vi "Begin.vi"(8 "error in":errorcluster) -> (0 "error out":errorcluster)   [LabVIEW 2017]
doc: "Called before other user functions, this VI is expected to open initial I/O refnums, load in file data, and do all program initialization. Notice that the <B>error out</B> terminal is simply used for data flow. Wiring it to other structures or subVIs ensures that this VI runs first."
uses:
  <vilib>/Rock Robotics/WPI/SafetyOutput/WPI_SafetyOutputConfigMenu.ctl
  <vilib>/Rock Robotics/WPI/Joystick/WPI_JoystickDeviceEnum.ctl
  <vilib>/Rock Robotics/WPI/DriverStation/WPI_DriverStationRobotMode2.ctl
  <vilib>/Rock Robotics/WPI/Solenoid/WPI_SolenoidChannel.ctl
  <vilib>/Rock Robotics/WPI/ThirdParty/Phoenix-LabVIEW/Motor Controller/Controls/CTRE_Phoenix_MotorControl_NeutralMode.ctl
  <vilib>/Rock Robotics/SystemInterfaces/DIO/FPGA_DIOChannel.ctl
  <vilib>/Rock Robotics/WPI/Solenoid/WPI_SolenoidValue.ctl
  <vilib>/Rock Robotics/Network Tables/NT Write String Array.vi
  <vilib>/Rock Robotics/WPI/Solenoid/WPI_SolenoidOpenDouble.vi
  Robot Global Data.vi
  <vilib>/Rock Robotics/WPI/Solenoid/WPI_SolenoidSetEnum.vi
  <vilib>/Rock Robotics/WPI/Counter/WPI_CounterDigitalInputToDigitalSource.vi
  <vilib>/Rock Robotics/WPI/ThirdParty/Phoenix-LabVIEW/Pigeon IMU/CTRE_PigeonIMU_Open_TalonSRX.vi
  <vilib>/Rock Robotics/WPI/RobotDrive/WPI_RobotDriveOpen2MotorWithExistingMotors.vi
  <vilib>/Rock Robotics/WPI/RobotDrive/WPI_RobotDriveOpen4MotorWithExistingMotors.vi
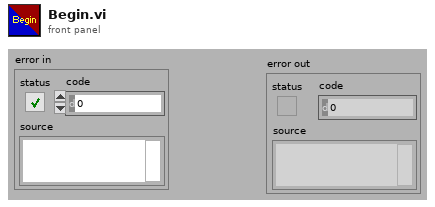
[diagram p1: front panel]
types:
  T1 = typedef "WPI_SolenoidValue.ctl" = enum16{"Off", "On", "Forward", "Reverse"}
  T2 = typedef "WPI_SolenoidChannel.ctl" = enum8{"Solenoid 0", "Solenoid 1", "Solenoid 2", "Solenoid 3", "Solenoid 4", "Solenoid 5", "Solenoid 6", "Solenoid 7", "Invalid"}
  T3 = typedef "FPGA_DIOChannel.ctl" = enum8{"DIO 0", "DIO 1", "DIO 2", "DIO 3", "DIO 4", "DIO 5", "DIO 6", "DIO 7", "DIO 8", "DIO 9", "DIO MXP 0", "DIO MXP 1", "DIO MXP 2", "DIO MXP 3", "DIO MXP 4", "DIO MXP 5", "DIO MXP 6", "DIO MXP 7", "DIO MXP 8", "DIO MXP 9", "DIO MXP 10", "DIO MXP 11", "DIO MXP 12", "DIO MXP 13", "DIO MXP 14", "DIO MXP 15", "SPI Port CS1", "SPI Port CS2", "SPI Port CS3", "SPI Port MISO", "SPI Port MOSI", "Invalid"}
  T4 = typedef "CTRE_Phoenix_MotorControl_NeutralMode.ctl" = enum8{"EEPROMSetting", "Override to Coast", "Override to Brake"}
  T5 = typedef "WPI_JoystickDeviceEnum.ctl" = enum16{"USB 0", "USB 1", "USB 2", "USB 3", "USB 4", "USB 5"}
  T6 = typedef "WPI_DriverStationRobotMode2.ctl" = enum16{"Autonomous Disabled", "Autonomous Enabled", "Teleop Disabled", "Teleop Enabled", "Disconnected", "Finish", "Test Disabled", "Test Enabled", "Emergency Stopped"}
  T7 = typedef "WPI_SafetyOutputConfigMenu.ctl" = enum16{"Enable", "Disable"}
  T8 = enum16{"FollowerType_PercentOutput", "FollowerType_AuxOutput1"}
  T9 = typedef "WPI_MotorControlDeviceRef.ctl" = cluster{"DeviceStatus":errorcluster, "Type":T10, "PWM":cluster{"PWM Channel":T11, "DeadBand":T12}, "CAN":cluster{"Device Number":u8, "SetOutput VI Ref":variant, "GetOutput VI Ref":variant, "Enable VI Ref":variant, "Disable VI Ref":variant, "Data":variant}, "Invert":bool, "DIO PWM":cluster{"PWM \"Enable\" Channel":T11, "DIOChannel":T3, "PWM Rate":dbl}}
  T10 = typedef "WPI_MotorControlType.ctl" = enum16{"PWM", "CAN", "DIO PWM"}
  T11 = typedef "FPGA_DIOPWMChannel.ctl" = enum8{"PWM 0", "PWM 1", "PWM 2", "PWM 3", "PWM 4", "PWM 5", "PWM 6", "PWM 7", "PWM 8", "PWM 9", "PWM MXP 0", "PWM MXP 1", "PWM MXP 2", "PWM MXP 3", "PWM MXP 4", "PWM MXP 5", "PWM MXP 6", "PWM MXP 7", "PWM MXP 8", "PWM MXP 9", "Invalid"}
  T12 = typedef "WPI_PWMDeadband.ctl" = cluster{"Name":string, "maxPositivePwm":i32, "minPositivePwm":i32, "centerPwm":i32, "maxNegativePwm":i32, "minNegativePwm":i32, "angularRange":u16}
  T13 = typedef "CTRE_PigeonIMU_DeviceRef.ctl" = cluster{"DeviceStatus":errorcluster, "Device Number":u8, "Type":T14, "Device ID":u32, "Handle":u64, "UsageFrame":u32, "Library Path":path}
  T14 = typedef "CTRE_PigeonIMU_ConnectionType.ctl" = u32
  T15 = typedef "WPI_RobotDriveDevRef.ctl" = cluster{"DevStatus":errorcluster, "Motors[]":T9[], "Square Inputs":bool, "Max Output":dbl}
  T16 = typedef "WPI_CompressorDevRef.ctl" = cluster{"DevStatus":errorcluster, "Pneumatics Control Module":u8}
  T17 = typedef "WPI_DigitalInputDevRef.ctl" = cluster{"DevStatus":errorcluster, "DIO Channel":T3}
  T18 = typedef "WPI_JoystickDevRef.ctl" = cluster{"Device":T5}
  T19 = typedef "FPGA_CounterEncoderSourceConvertionLVSourceType.ctl" = cluster{"DevStatus":errorcluster, "AnalogTriggerMode?":bool, "DigitalMode":cluster{"DIO Channel":T20}, "AnalogTriggerMode":cluster{"AnalogTriggerIndex":T21, "OutputType":T22}}
  T20 = typedef "FPGA_DIODigitalSourceChannel.ctl" = enum8{"DIO 0", "DIO 1", "DIO 2", "DIO 3", "DIO 4", "DIO 5", "DIO 6", "DIO 7", "DIO 8", "DIO 9", "DIO MXP 0", "DIO MXP 1", "DIO MXP 2", "DIO MXP 3", "DIO MXP 4", "DIO MXP 5", "DIO MXP 6", "DIO MXP 7", "DIO MXP 8", "DIO MXP 9", "DIO MXP 10", "DIO MXP 11", "DIO MXP 12", "DIO MXP 13", "DIO MXP 14", "DIO MXP 15", "Disabled"}
  T21 = typedef "FPGA_AnalogTriggerIndex.ctl" = enum8{"Trig 0", "Trig 1", "Trig 2", "Trig 3", "Trig 4", "Trig 5", "Trig 6", "Trig 7", "Invalid"}
  T22 = typedef "FPGA_AnalogTriggerOutType.ctl" = enum16{"InWindow", "TriggerState", "Rising", "Falling"}
  T23 = typedef "WPI_SolenoidDevRef.ctl" = cluster{"DevStatus":errorcluster, "Pneumatics Control Module":u8, "Forward Solenoid Channel":T2, "Reverse Solenoid Channel":T2}
  T24 = typedef "WPI_EncoderDevRef.ctl" = cluster{"DevStatus":errorcluster, "EncoderIndex":T25, "CounterIndex":T26, "DistancePerCount":dbl, "Decoding Type":T27}
  T25 = typedef "FPGA_EncoderIdx.ctl" = enum8{"Enc 0", "Enc 1", "Enc 2", "Enc 3", "Enc 4", "Enc 5", "Enc 6", "Enc 7", "Invalid"}
  T26 = typedef "FPGA_CounterCtrSystemIndex.ctl" = enum8{"Ctr 0", "Ctr 1", "Ctr 2", "Ctr 3", "Ctr 4", "Ctr 5", "Ctr 6", "Ctr 7", "Invalid"}
  T27 = typedef "WPI_EncoderType.ctl" = enum16{"1x", "2x", "4x"}
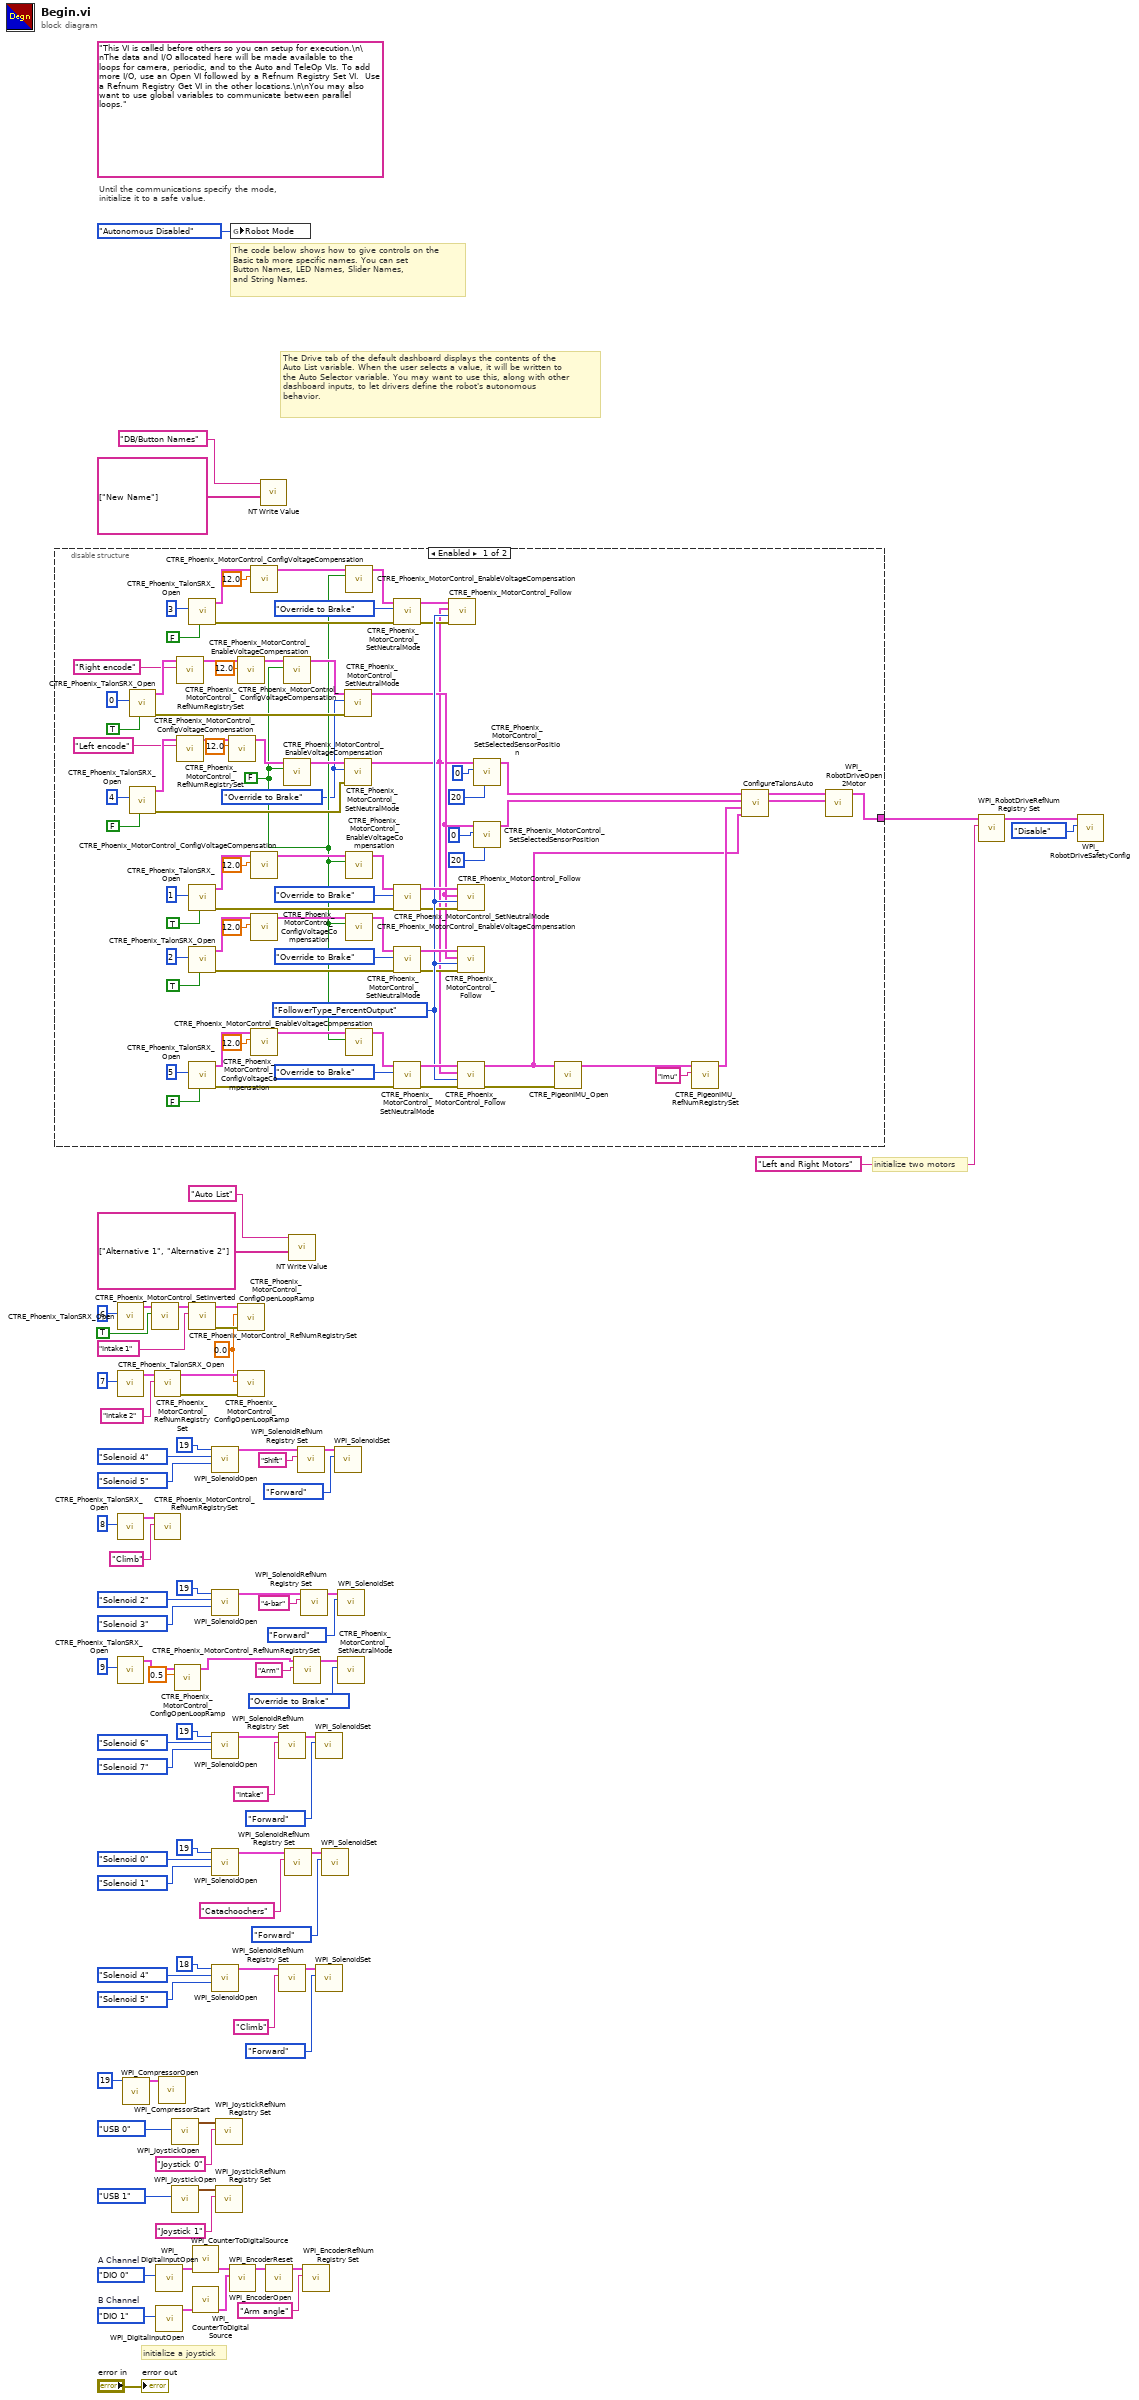
[diagram p0: block diagram]
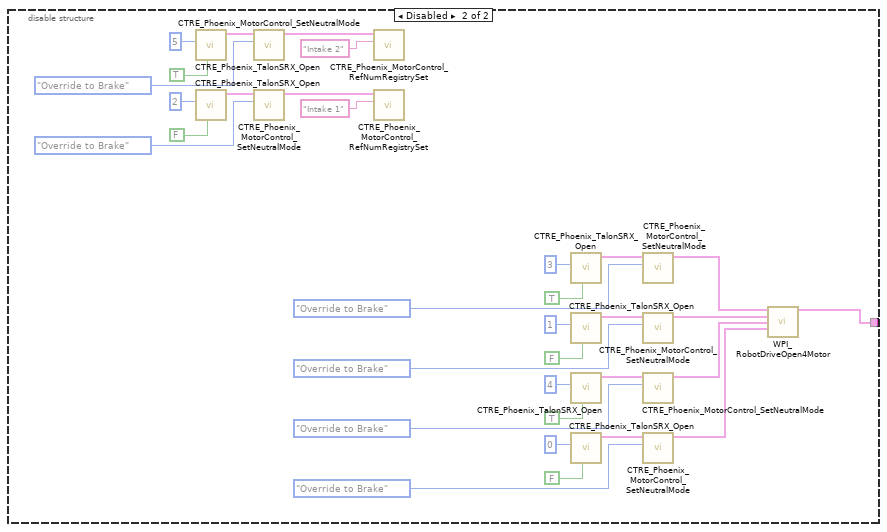
[diagram p2: hidden frame]
diagram:
  w2 = 0.0 ("secondsFromNeutralToFull")
  w35 = FPGA_DIOChannel."DIO 1"  # B Channel
  w34 = FPGA_DIOChannel."DIO 0"  # A Channel
  (unwired) "This VI is called before others so you can setup for execution.\n\nThe data and I/O allocated here will be made available to the loops for camera, periodic, and to the Auto and TeleOp VIs. To add more I/O, use an Open VI followed by a Refnum Registry Set VI.  Use a Refnum Registry Get VI in the other locations.\n\nYou may also want to use global variables to communicate between parallel loops."
  # "The Drive tab of the default dashboard displays the contents of the\nAuto List variable. When the user selects a value, it will be written to\nthe Auto Selector variable. You may want to use this, along with other\ndashboard inputs, to let drivers define the robot's autonomous\nbehavior."
  # "The code below shows how to give controls on the\nBasic tab more specific names. You can set\nButton Names, LED Names, Slider Names,\nand String Names."
  # "initialize a joystick"
  # "Until the communications specify the mode,\ninitialize it to a safe value."
  # "initialize two motors"
  n1 = disable-structure shown="Enabled" {
    disable-tunnel: [w134 w175] -> w1
    frame Enabled {
      w102 = FALSE ("Enable Voltage Compensation?")
      w129 = T8."FollowerType_PercentOutput" ("FollowerType")
      w92 = CTRE_Phoenix_MotorControl_NeutralMode."Override to Brake" ("Motor Control Neutral Mode")
      n2 = call <vilib>:"CTRE_Phoenix_TalonSRX_Open.vi"("Invert"=TRUE, "Device Number"=u8 0) -> ("error out"=w147:errorcluster, "CAN Talon SRX Ref"=w98:T9)  [unwired: 8 in]
      n3 = call <vilib>:"CTRE_Phoenix_TalonSRX_Open.vi"("Invert"=FALSE, "Device Number"=u8 4) -> ("error out"=w161:errorcluster, "CAN Talon SRX Ref"=w96:T9)  [unwired: 8 in]
      n4 = call <vilib>:"CTRE_Phoenix_MotorControl_RefNumRegistrySet.vi"("refnum name"="Right encode", "PhoenixMotorControlDevRef"=w98) -> ("PhoenixMotorControlDevRef"=w97:T9)  [unwired: 8 in, 1 out]
      n5 = call <vilib>:"CTRE_Phoenix_MotorControl_RefNumRegistrySet.vi"("refnum name"="Left encode", "PhoenixMotorControlDevRef"=w96) -> ("PhoenixMotorControlDevRef"=w95:T9)  [unwired: 8 in, 1 out]
      n6 = call <vilib>:"CTRE_Phoenix_TalonSRX_Open.vi"("Invert"=FALSE, "Device Number"=u8 3) -> ("error out"=w162:errorcluster, "CAN Talon SRX Ref"=w123:T9)  [unwired: 8 in]
      n7 = call <vilib>:"CTRE_Phoenix_TalonSRX_Open.vi"("Invert"=TRUE, "Device Number"=u8 1) -> ("error out"=w155:errorcluster, "CAN Talon SRX Ref"=w120:T9)  [unwired: 8 in]
      n8 = call <vilib>:"CTRE_Phoenix_TalonSRX_Open.vi"("Invert"=TRUE, "Device Number"=u8 2) -> ("error out"=w154:errorcluster, "CAN Talon SRX Ref"=w121:T9)  [unwired: 8 in]
      n9 = call <vilib>:"CTRE_Phoenix_TalonSRX_Open.vi"("Invert"=FALSE, "Device Number"=u8 5) -> ("error out"=w146:errorcluster, "CAN Talon SRX Ref"=w122:T9)  [unwired: 8 in]
      n10 = call <vilib>:"CTRE_Phoenix_MotorControl_ConfigVoltageCompensation.vi"("Saturation Voltage"=12.0, "PhoenixMotorControlDevRef"=w95) -> ("PhoenixMotorControlDevRef"=w106:T9)  [unwired: 8 in, 1 out]
      n11 = call <vilib>:"CTRE_Phoenix_MotorControl_ConfigVoltageCompensation.vi"("Saturation Voltage"=12.0, "PhoenixMotorControlDevRef"=w97) -> ("PhoenixMotorControlDevRef"=w108:T9)  [unwired: 8 in, 1 out]
      n12 = call <vilib>:"CTRE_Phoenix_MotorControl_ConfigVoltageCompensation.vi"("Saturation Voltage"=12.0, "PhoenixMotorControlDevRef"=w123) -> ("PhoenixMotorControlDevRef"=w114:T9)  [unwired: 8 in, 1 out]
      n13 = call <vilib>:"CTRE_Phoenix_MotorControl_ConfigVoltageCompensation.vi"("Saturation Voltage"=12.0, "PhoenixMotorControlDevRef"=w120) -> ("PhoenixMotorControlDevRef"=w110:T9)  [unwired: 8 in, 1 out]
      n14 = call <vilib>:"CTRE_Phoenix_MotorControl_ConfigVoltageCompensation.vi"("Saturation Voltage"=12.0, "PhoenixMotorControlDevRef"=w121) -> ("PhoenixMotorControlDevRef"=w112:T9)  [unwired: 8 in, 1 out]
      n15 = call <vilib>:"CTRE_Phoenix_MotorControl_ConfigVoltageCompensation.vi"("Saturation Voltage"=12.0, "PhoenixMotorControlDevRef"=w122) -> ("PhoenixMotorControlDevRef"=w104:T9)  [unwired: 8 in, 1 out]
      n16 = call <vilib>:"CTRE_Phoenix_MotorControl_EnableVoltageCompensation.vi"("Enable Voltage Compensation?"=w102, "PhoenixMotorControlDevRef"=w108) -> ("PhoenixMotorControlDevRef"=w107:T9)  [unwired: 8 in, 1 out]
      n17 = call <vilib>:"CTRE_Phoenix_MotorControl_EnableVoltageCompensation.vi"("Enable Voltage Compensation?"=w102, "PhoenixMotorControlDevRef"=w106) -> ("PhoenixMotorControlDevRef"=w105:T9)  [unwired: 8 in, 1 out]
      n18 = call <vilib>:"CTRE_Phoenix_MotorControl_SetNeutralMode.vi"("error in (no error)"=w147, "Motor Control Neutral Mode"=w92, "PhoenixMotorControlDevRef"=w107) -> ("PhoenixMotorControlDevRef"=w101:T9)  [unwired: 7 in, 1 out]
      n19 = call <vilib>:"CTRE_Phoenix_MotorControl_SetNeutralMode.vi"("error in (no error)"=w161, "Motor Control Neutral Mode"=w92, "PhoenixMotorControlDevRef"=w105) -> ("PhoenixMotorControlDevRef"=w100:T9)  [unwired: 7 in, 1 out]
      n20 = call <vilib>:"CTRE_Phoenix_MotorControl_EnableVoltageCompensation.vi"("Enable Voltage Compensation?"=w102, "PhoenixMotorControlDevRef"=w114) -> ("PhoenixMotorControlDevRef"=w113:T9)  [unwired: 8 in, 1 out]
      n21 = call <vilib>:"CTRE_Phoenix_MotorControl_EnableVoltageCompensation.vi"("Enable Voltage Compensation?"=w102, "PhoenixMotorControlDevRef"=w110) -> ("PhoenixMotorControlDevRef"=w109:T9)  [unwired: 8 in, 1 out]
      n22 = call <vilib>:"CTRE_Phoenix_MotorControl_EnableVoltageCompensation.vi"("Enable Voltage Compensation?"=w102, "PhoenixMotorControlDevRef"=w112) -> ("PhoenixMotorControlDevRef"=w111:T9)  [unwired: 8 in, 1 out]
      n23 = call <vilib>:"CTRE_Phoenix_MotorControl_EnableVoltageCompensation.vi"("Enable Voltage Compensation?"=w102, "PhoenixMotorControlDevRef"=w104) -> ("PhoenixMotorControlDevRef"=w103:T9)  [unwired: 8 in, 1 out]
      n24 = call <vilib>:"CTRE_Phoenix_MotorControl_SetNeutralMode.vi"("error in (no error)"=w162, "Motor Control Neutral Mode"=CTRE_Phoenix_MotorControl_NeutralMode."Override to Brake", "PhoenixMotorControlDevRef"=w113) -> ("error out"=w128:errorcluster, "PhoenixMotorControlDevRef"=w133:T9)  [unwired: 7 in]
      n25 = call <vilib>:"CTRE_Phoenix_MotorControl_SetNeutralMode.vi"("error in (no error)"=w155, "Motor Control Neutral Mode"=CTRE_Phoenix_MotorControl_NeutralMode."Override to Brake", "PhoenixMotorControlDevRef"=w109) -> ("error out"=w126:errorcluster, "PhoenixMotorControlDevRef"=w131:T9)  [unwired: 7 in]
      n26 = call <vilib>:"CTRE_Phoenix_MotorControl_SetNeutralMode.vi"("error in (no error)"=w154, "Motor Control Neutral Mode"=CTRE_Phoenix_MotorControl_NeutralMode."Override to Brake", "PhoenixMotorControlDevRef"=w111) -> ("error out"=w125:errorcluster, "PhoenixMotorControlDevRef"=w130:T9)  [unwired: 7 in]
      n27 = call <vilib>:"CTRE_Phoenix_MotorControl_SetNeutralMode.vi"("error in (no error)"=w146, "Motor Control Neutral Mode"=CTRE_Phoenix_MotorControl_NeutralMode."Override to Brake", "PhoenixMotorControlDevRef"=w103) -> ("error out"=w127:errorcluster, "PhoenixMotorControlDevRef"=w132:T9)  [unwired: 7 in]
      n28 = call <vilib>:"CTRE_Phoenix_MotorControl_Follow.vi"("error in (no error)"=w128, "FollowerType"=w129, "Master Controller to Follow"=w100, "PhoenixMotorControlDevRef"=w133) -> ()  [unwired: 6 in, 2 out]
      n29 = call <vilib>:"CTRE_Phoenix_MotorControl_Follow.vi"("error in (no error)"=w126, "FollowerType"=w129, "Master Controller to Follow"=w101, "PhoenixMotorControlDevRef"=w131) -> ()  [unwired: 6 in, 2 out]
      n30 = call <vilib>:"CTRE_Phoenix_MotorControl_Follow.vi"("error in (no error)"=w125, "FollowerType"=w129, "Master Controller to Follow"=w101, "PhoenixMotorControlDevRef"=w130) -> ()  [unwired: 6 in, 2 out]
      n31 = call <vilib>:"CTRE_Phoenix_MotorControl_Follow.vi"("error in (no error)"=w127, "FollowerType"=w129, "Master Controller to Follow"=w100, "PhoenixMotorControlDevRef"=w132) -> ("error out"=w124:errorcluster, "PhoenixMotorControlDevRef"=w87:T9)  [unwired: 6 in]
      n32 = call <vilib>:"CTRE_Phoenix_MotorControl_SetSelectedSensorPosition.vi"("timeoutMs"=u32 20, "New Sensor Position"=0, "PhoenixMotorControlDevRef"=w100) -> ("PhoenixMotorControlDevRef"=w89:T9)  [unwired: 7 in, 1 out]
      n33 = call <vilib>:"CTRE_Phoenix_MotorControl_SetSelectedSensorPosition.vi"("timeoutMs"=u32 20, "New Sensor Position"=0, "PhoenixMotorControlDevRef"=w101) -> ("PhoenixMotorControlDevRef"=w86:T9)  [unwired: 7 in, 1 out]
      n34 = call-poly <vilib>:"CTRE_PigeonIMU_Open.vi"("error in"=w124, "CAN Talon SRX Ref"=w87) -> ("PigeonIMUDevRef"=w136:T13)  [unwired: 8 in, 1 out]
      n35 = call <vilib>:"CTRE_PigeonIMU_RefNumRegistrySet.vi"("refnum name"="imu", "PigeonIMUDevRef"=w136) -> ("PigeonIMUDevRef"=w88:T13)  [unwired: 8 in, 1 out]
      n36 = call "ConfigureTalonsAuto.vi"("Pigeon Talon"=w87, "Pigeon"=w88, "Right Side"=w86, "Left Side"=w89) -> ("Right Side"=w90:T9, "Left Side"=w91:T9)  [unwired: 6 in]
      n37 = call-poly <vilib>:"WPI_RobotDriveOpen2Motor.vi"("Right Motor Dev Ref"=w90, "Left Motor Dev Ref"=w91) -> ("RobotDriveDevRef"=w134:T15)  [unwired: 8 in, 1 out]
    }
    frame Disabled {
      n38 = call <vilib>:"CTRE_Phoenix_TalonSRX_Open.vi"("Invert"=TRUE, "Device Number"=u8 5) -> ("CAN Talon SRX Ref"=w172:T9)  [unwired: 8 in, 1 out]
      n39 = call <vilib>:"CTRE_Phoenix_TalonSRX_Open.vi"("Invert"=FALSE, "Device Number"=u8 2) -> ("CAN Talon SRX Ref"=w171:T9)  [unwired: 8 in, 1 out]
      n40 = call <vilib>:"CTRE_Phoenix_MotorControl_SetNeutralMode.vi"("Motor Control Neutral Mode"=CTRE_Phoenix_MotorControl_NeutralMode."Override to Brake", "PhoenixMotorControlDevRef"=w172) -> ("PhoenixMotorControlDevRef"=w174:T9)  [unwired: 8 in, 1 out]
      n41 = call <vilib>:"CTRE_Phoenix_MotorControl_SetNeutralMode.vi"("Motor Control Neutral Mode"=CTRE_Phoenix_MotorControl_NeutralMode."Override to Brake", "PhoenixMotorControlDevRef"=w171) -> ("PhoenixMotorControlDevRef"=w173:T9)  [unwired: 8 in, 1 out]
      n42 = call <vilib>:"CTRE_Phoenix_MotorControl_RefNumRegistrySet.vi"("refnum name"="Intake 2", "PhoenixMotorControlDevRef"=w174) -> ()  [unwired: 8 in, 2 out]
      n43 = call <vilib>:"CTRE_Phoenix_MotorControl_RefNumRegistrySet.vi"("refnum name"="Intake 1", "PhoenixMotorControlDevRef"=w173) -> ()  [unwired: 8 in, 2 out]
      n44 = call <vilib>:"CTRE_Phoenix_TalonSRX_Open.vi"("Invert"=TRUE, "Device Number"=u8 3) -> ("CAN Talon SRX Ref"=w195:T9)  [unwired: 8 in, 1 out]
      n45 = call <vilib>:"CTRE_Phoenix_TalonSRX_Open.vi"("Invert"=FALSE, "Device Number"=u8 1) -> ("CAN Talon SRX Ref"=w190:T9)  [unwired: 8 in, 1 out]
      n46 = call <vilib>:"CTRE_Phoenix_TalonSRX_Open.vi"("Invert"=TRUE, "Device Number"=u8 4) -> ("CAN Talon SRX Ref"=w192:T9)  [unwired: 8 in, 1 out]
      n47 = call <vilib>:"CTRE_Phoenix_TalonSRX_Open.vi"("Invert"=FALSE, "Device Number"=u8 0) -> ("CAN Talon SRX Ref"=w188:T9)  [unwired: 8 in, 1 out]
      n48 = call <vilib>:"CTRE_Phoenix_MotorControl_SetNeutralMode.vi"("Motor Control Neutral Mode"=CTRE_Phoenix_MotorControl_NeutralMode."Override to Brake", "PhoenixMotorControlDevRef"=w195) -> ("PhoenixMotorControlDevRef"=w193:T9)  [unwired: 8 in, 1 out]
      n49 = call <vilib>:"CTRE_Phoenix_MotorControl_SetNeutralMode.vi"("Motor Control Neutral Mode"=CTRE_Phoenix_MotorControl_NeutralMode."Override to Brake", "PhoenixMotorControlDevRef"=w190) -> ("PhoenixMotorControlDevRef"=w186:T9)  [unwired: 8 in, 1 out]
      n50 = call <vilib>:"CTRE_Phoenix_MotorControl_SetNeutralMode.vi"("Motor Control Neutral Mode"=CTRE_Phoenix_MotorControl_NeutralMode."Override to Brake", "PhoenixMotorControlDevRef"=w192) -> ("PhoenixMotorControlDevRef"=w185:T9)  [unwired: 8 in, 1 out]
      n51 = call <vilib>:"CTRE_Phoenix_MotorControl_SetNeutralMode.vi"("Motor Control Neutral Mode"=CTRE_Phoenix_MotorControl_NeutralMode."Override to Brake", "PhoenixMotorControlDevRef"=w188) -> ("PhoenixMotorControlDevRef"=w184:T9)  [unwired: 8 in, 1 out]
      n52 = call-poly <vilib>:"WPI_RobotDriveOpen4Motor.vi"("Rear Left Motor Dev Ref"=w193, "Rear Right Motor Dev Ref"=w186, "Front Left Motor Dev Ref"=w185, "Front Right Motor Dev Ref"=w184) -> ("RobotDriveDevRef"=w175:T15)  [unwired: 10 in, 1 out]
    }
  }
  n53 = call <vilib>:"CTRE_Phoenix_TalonSRX_Open.vi"("Device Number"=u8 6) -> ("CAN Talon SRX Ref"=w19:T9)  [unwired: 9 in, 1 out]
  n54 = call <vilib>:"CTRE_Phoenix_TalonSRX_Open.vi"("Device Number"=u8 7) -> ("CAN Talon SRX Ref"=w59:T9)  [unwired: 9 in, 1 out]
  n55 = call <vilib>:"CTRE_Phoenix_TalonSRX_Open.vi"("Device Number"=u8 8) -> ("CAN Talon SRX Ref"=w40:T9)  [unwired: 9 in, 1 out]
  n56 = call <vilib>:"CTRE_Phoenix_TalonSRX_Open.vi"("Device Number"=u8 9) -> ("CAN Talon SRX Ref"=w9:T9)  [unwired: 9 in, 1 out]
  n57 = call <vilib>:"WPI_CompressorOpen.vi"("Pneumatics Control Module (0)"=u8 19) -> ("CompressorDevRef"=w73:T16)  [unwired: 13 in, 1 out]
  n58 = call <vilib>:"CTRE_Phoenix_MotorControl_SetInverted.vi"("Invert?"=TRUE, "PhoenixMotorControlDevRef"=w19) -> ("PhoenixMotorControlDevRef"=w18:T9)  [unwired: 8 in, 1 out]
  n59 = call <vilib>:"CTRE_Phoenix_MotorControl_RefNumRegistrySet.vi"("refnum name"="Intake 2", "PhoenixMotorControlDevRef"=w59) -> ("error out"=w4:errorcluster, "PhoenixMotorControlDevRef"=w3:T9)  [unwired: 8 in]
  n60 = call <vilib>:"CTRE_Phoenix_MotorControl_RefNumRegistrySet.vi"("refnum name"="Climb", "PhoenixMotorControlDevRef"=w40) -> ()  [unwired: 8 in, 2 out]
  n61 = call <vilib>:"WPI_DigitalInputOpen.vi"("DIO Channel"=w34) -> ("DigitalInputDevRef"=w31:T17)  [unwired: 1 in, 9 out]
  n62 = call <vilib>:"WPI_DigitalInputOpen.vi"("DIO Channel"=w35) -> ("DigitalInputDevRef"=w32:T17)  [unwired: 1 in, 9 out]
  n63 = call <vilib>:"WPI_CompressorStart.vi"("CompressorDevRef"=w73) -> ()  [unwired: 9 in, 2 out]
  n64 = call <vilib>:"WPI_JoystickOpen.vi"("JoystickDevice"=WPI_JoystickDeviceEnum."USB 0") -> ("JoystickDevRef"=w81:T18)  [unwired: 10 in]
  n65 = call <vilib>:"WPI_JoystickOpen.vi"("JoystickDevice"=WPI_JoystickDeviceEnum."USB 1") -> ("JoystickDevRef"=w65:T18)  [unwired: 10 in]
  n66 = call <vilib>:"CTRE_Phoenix_MotorControl_ConfigOpenLoopRamp.vi"("secondsFromNeutralToFull"=0.5, "PhoenixMotorControlDevRef"=w9) -> ("PhoenixMotorControlDevRef"=w8:T9)  [unwired: 8 in, 1 out]
  n67 = call <vilib>:"CTRE_Phoenix_MotorControl_RefNumRegistrySet.vi"("refnum name"="Intake 1", "PhoenixMotorControlDevRef"=w18) -> ("error out"=w6:errorcluster, "PhoenixMotorControlDevRef"=w5:T9)  [unwired: 8 in]
  n68 = call-poly <vilib>:"WPI_CounterToDigitalSource.vi"("DigitalInputDevRef"=w31) -> ("Digital Source"=w30:T19)  [unwired: 6 out]
  n69 = call-poly <vilib>:"WPI_CounterToDigitalSource.vi"("DigitalInputDevRef"=w32) -> ("Digital Source"=w33:T19)  [unwired: 6 out]
  n70 = call-poly <vilib>:"WPI_SolenoidOpen.vi"("Reverse Solenoid Channel"=WPI_SolenoidChannel."Solenoid 5", "Forward Solenoid Channel"=WPI_SolenoidChannel."Solenoid 4", "Pneumatics Control Module (0)"=u8 19) -> ("SolenoidDevRef"=w69:T23)  [unwired: 7 in, 1 out]
  n71 = call-poly <vilib>:"WPI_SolenoidOpen.vi"("Reverse Solenoid Channel"=WPI_SolenoidChannel."Solenoid 3", "Forward Solenoid Channel"=WPI_SolenoidChannel."Solenoid 2", "Pneumatics Control Module (0)"=u8 19) -> ("SolenoidDevRef"=w53:T23)  [unwired: 7 in, 1 out]
  n72 = call-poly <vilib>:"WPI_SolenoidOpen.vi"("Reverse Solenoid Channel"=WPI_SolenoidChannel."Solenoid 7", "Forward Solenoid Channel"=WPI_SolenoidChannel."Solenoid 6", "Pneumatics Control Module (0)"=u8 19) -> ("SolenoidDevRef"=w46:T23)  [unwired: 7 in, 1 out]
  n73 = call-poly <vilib>:"WPI_SolenoidOpen.vi"("Reverse Solenoid Channel"=WPI_SolenoidChannel."Solenoid 1", "Forward Solenoid Channel"=WPI_SolenoidChannel."Solenoid 0", "Pneumatics Control Module (0)"=u8 19) -> ("SolenoidDevRef"=w23:T23)  [unwired: 7 in, 1 out]
  n74 = call-poly <vilib>:"WPI_SolenoidOpen.vi"("Reverse Solenoid Channel"=WPI_SolenoidChannel."Solenoid 5", "Forward Solenoid Channel"=WPI_SolenoidChannel."Solenoid 4", "Pneumatics Control Module (0)"=u8 18) -> ("SolenoidDevRef"=w13:T23)  [unwired: 7 in, 1 out]
  n75 = call <vilib>:"WPI_JoystickRefNum Registry Set.vi"("refnum name"="Joystick 0", "JoystickDevRef"=w81) -> ()  [unwired: 8 in, 2 out]
  n76 = call <vilib>:"WPI_JoystickRefNum Registry Set.vi"("refnum name"="Joystick 1", "JoystickDevRef"=w65) -> ()  [unwired: 8 in, 2 out]
  n77 = call <vilib>:"WPI_EncoderOpen.vi"("BSource"=w33, "ASource"=w30) -> ("EncoderDevRef"=w29:T24)  [unwired: 6 in, 3 out]
  n78 = global write "Robot Global Data.vi" "Robot Mode"(WPI_DriverStationRobotMode2."Autonomous Disabled" ("Robot Mode")) -> ()
  n79 = call <vilib>:"CTRE_Phoenix_MotorControl_ConfigOpenLoopRamp.vi"("error in (no error)"=w6, "secondsFromNeutralToFull"=w2, "PhoenixMotorControlDevRef"=w5) -> ()  [unwired: 7 in, 2 out]
  n80 = call <vilib>:"CTRE_Phoenix_MotorControl_ConfigOpenLoopRamp.vi"("error in (no error)"=w4, "secondsFromNeutralToFull"=w2, "PhoenixMotorControlDevRef"=w3) -> ()  [unwired: 7 in, 2 out]
  n81 = call-poly <vilib>:"NT Write Value.vi"("String Array"=string[] ["New Name"], "Name"="DB/Button Names") -> ()  [unwired: 9 in, 1 out]
  n82 = call <vilib>:"WPI_EncoderReset.vi"("EncoderDevRef"=w29) -> ("EncoderDevRef"=w28:T24)  [unwired: 9 in, 1 out]
  n83 = call <vilib>:"WPI_SolenoidRefNum Registry Set.vi"("refnum name"="Intake", "SolenoidDevRef"=w46) -> ("SolenoidDevRef"=w44:T23)  [unwired: 8 in, 1 out]
  n84 = call <vilib>:"WPI_SolenoidRefNum Registry Set.vi"("refnum name"="Climb", "SolenoidDevRef"=w13) -> ("SolenoidDevRef"=w15:T23)  [unwired: 8 in, 1 out]
  n85 = call <vilib>:"WPI_SolenoidRefNum Registry Set.vi"("refnum name"="Catachoochers", "SolenoidDevRef"=w23) -> ("SolenoidDevRef"=w21:T23)  [unwired: 8 in, 1 out]
  n86 = call-poly <vilib>:"NT Write Value.vi"("String Array"=string[] ["Alternative 1", "Alternative 2"], "Name"="Auto List") -> ()  [unwired: 9 in, 1 out]
  n87 = call <vilib>:"CTRE_Phoenix_MotorControl_RefNumRegistrySet.vi"("refnum name"="Arm", "PhoenixMotorControlDevRef"=w8) -> ("PhoenixMotorControlDevRef"=w37:T9)  [unwired: 8 in, 1 out]
  n88 = call <vilib>:"WPI_SolenoidRefNum Registry Set.vi"("refnum name"="Shift", "SolenoidDevRef"=w69) -> ("SolenoidDevRef"=w63:T23)  [unwired: 8 in, 1 out]
  n89 = call <vilib>:"WPI_SolenoidRefNum Registry Set.vi"("refnum name"="4-bar", "SolenoidDevRef"=w53) -> ("SolenoidDevRef"=w55:T23)  [unwired: 8 in, 1 out]
  n90 = call <vilib>:"WPI_EncoderRefNum Registry Set.vi"("refnum name"="Arm angle", "EncoderDevRef"=w28) -> ()  [unwired: 8 in, 2 out]
  n91 = call-poly <vilib>:"WPI_SolenoidSet.vi"("Value"=WPI_SolenoidValue."Forward", "SolenoidDevRef"=w44) -> ()  [unwired: 8 in, 2 out]
  n92 = call-poly <vilib>:"WPI_SolenoidSet.vi"("Value"=WPI_SolenoidValue."Forward", "SolenoidDevRef"=w15) -> ()  [unwired: 8 in, 2 out]
  n93 = call-poly <vilib>:"WPI_SolenoidSet.vi"("Value"=WPI_SolenoidValue."Forward", "SolenoidDevRef"=w21) -> ()  [unwired: 8 in, 2 out]
  n94 = call-poly <vilib>:"WPI_SolenoidSet.vi"("Value"=WPI_SolenoidValue."Forward", "SolenoidDevRef"=w63) -> ()  [unwired: 8 in, 2 out]
  n95 = call-poly <vilib>:"WPI_SolenoidSet.vi"("Value"=WPI_SolenoidValue."Forward", "SolenoidDevRef"=w55) -> ()  [unwired: 8 in, 2 out]
  n96 = call <vilib>:"CTRE_Phoenix_MotorControl_SetNeutralMode.vi"("Motor Control Neutral Mode"=CTRE_Phoenix_MotorControl_NeutralMode."Override to Brake", "PhoenixMotorControlDevRef"=w37) -> ()  [unwired: 8 in, 2 out]
  n97 = call <vilib>:"WPI_RobotDriveRefNum Registry Set.vi"("refnum name"="Left and Right Motors", "RobotDriveDevRef"=w1) -> ("RobotDriveDevRef"=w84:T15)  [unwired: 2 in, 7 out]
  n98 = call <vilib>:"WPI_RobotDriveSafetyConfig.vi"("mode"=WPI_SafetyOutputConfigMenu."Disable", "RobotDriveDevRef"=w84) -> ()  [unwired: 8 in, 2 out]
  "error out" <- "error in"
